vi "Shooting Managment.vi"(0 "Start Shooting Procedure":bool) -> (1 "Disable Stack Ordering":bool, 2 "Is Shooting?":bool)   [LabVIEW 2012]
uses:
  BotStatus.vi
panel:
  # "ADD Override!!!!!!!!!!!!!!!!!!!!!!!!"
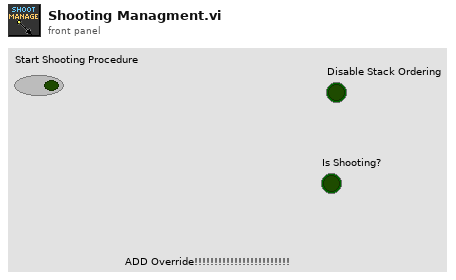
[diagram p1: front panel]
types:
  T1 = cluster{"Middle":bool, "Cannon":bool, "InFlipper":bool, "FlipperAtPlace":bool, "Bottom":bool, "FrisbeeDirection":bool}
  T2 = typedef "WPI_MotorControlDeviceRef.ctl" = cluster{"DeviceStatus":errorcluster, "Type":enum16{"PWM", "CAN"}, "PWM":cluster{"Digital Module":T3, "PWM Channel":T4, "DeadBand":T5}, "CAN":cluster{"Device Number":u8, "Control Mode":T6, "Semaphore":T7, "Max Vout":dbl}, "Invert":bool, "TransformRef":T8, "InvTransformRef":T8}
  T3 = typedef "FPGA_TypedefDigitalModule.ctl" = enum16{"Digital Module 1", "Digital Module 2"}
  T4 = typedef "FPGA_DIOPWMChannel.ctl" = enum8{"PWM 1", "PWM 2", "PWM 3", "PWM 4", "PWM 5", "PWM 6", "PWM 7", "PWM 8", "PWM 9", "PWM 10", "Invalid"}
  T5 = typedef "WPI_PWMDeadband.ctl" = cluster{"Name":string, "maxPositivePwm":i32, "minPositivePwm":i32, "centerPwm":i32, "maxNegativePwm":i32, "minNegativePwm":i32, "angularRange":u16}
  T6 = typedef "WPI_CANJaguar_ControlMode.ctl" = enum8{"Percent VBus", "Current", "Speed", "Position", "Voltage"}
  T7 = typedef "Semaphore RefNum" = refnum<k1>
  T8 = typedef "WPI_PWMTransform_ConPane.ctl" = refnum<vi>
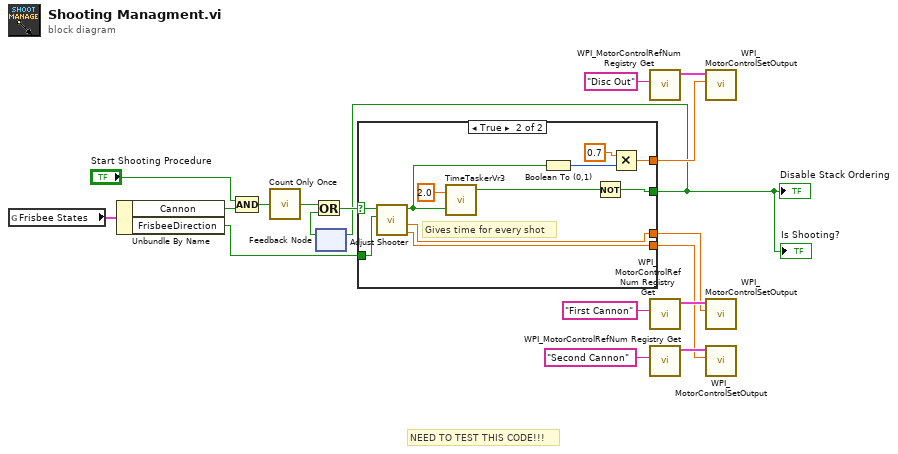
[diagram p0: block diagram]
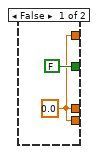
[diagram p2: hidden frame]
diagram:
  # "NEED TO TEST THIS CODE!!!"
  n1 = global read "BotStatus.vi" "Frisbee States"() -> (w5:T1)
  n2 = Unbundle By Name(w5) -> ("Cannon"=w3:bool, "FrisbeeDirection"=w4:bool)
  n3 = Compound Arithmetic op=AND("Start Shooting Procedure", w3) -> (w2:bool)
  n4 = call "Count Only Once.vi"("InValue"=w2) -> ("Result"=w17:bool)
  n5 = feedback #1() -> (w16:bool)  [unwired: 1 in]
  n6 = Or(x=w17, y=w16) -> (x .or. y?=w18:bool)
  n7 = case shown="True" w18 {
    selector: w18 -> [_ w24]
    tunnel: [FALSE ("READY!") w25] -> w1
    tunnel: [w19 w29] -> w13
    tunnel: [w19 w23] -> w8
    tunnel: [w19 w22] -> w7
    tunnel: w4 -> [_ w21]
    frame False {
      w19 = 0.0
    }
    frame True {
      # "Gives time for every shot"
      n8 = call "Adjust Shooter.vi"("Upside Down?"=w21, "Start to Adjust"=w24) -> ("Second Cannon"=w22:dbl, "First Cannon"=w23:dbl, "READY!"=w27:bool)  [unwired: 2 in, 1 out]
      n9 = call "TimeTaskerVr3.vi"("Delay(sec)"=2.0, "Start Counting?"=w27) -> ("TimePast?"=w26:bool)  [unwired: 2 out]
      n10 = Boolean To (0,1)(Boolean=w27) -> (0, 1=w31:i16)
      n11 = Not(x=w26) -> (.not. x?=w25:bool)
      n12 = Multiply(x=0.7, y=w31) -> (x*y=w29:dbl)
    }
  }
  "Disable Stack Ordering" <- w1
  "Is Shooting?" <- w1
  n13 = feedback-in #1(w1) -> ()
  n14 = call <vilib>:"WPI_MotorControlRefNum Registry Get.vi"("refnum name"="Disc Out") -> ("MotorControlDevRef"=w15:T2)  [unwired: 9 in, 1 out]
  n15 = call <vilib>:"WPI_MotorControlRefNum Registry Get.vi"("refnum name"="First Cannon") -> ("MotorControlDevRef"=w12:T2)  [unwired: 9 in, 1 out]
  n16 = call <vilib>:"WPI_MotorControlRefNum Registry Get.vi"("refnum name"="Second Cannon") -> ("MotorControlDevRef"=w11:T2)  [unwired: 9 in, 1 out]
  n17 = call <vilib>:"WPI_MotorControlSetOutput.vi"("Output"=w13, "MotorControlDevRef"=w15) -> ()  [unwired: 7 in, 3 out]
  n18 = call <vilib>:"WPI_MotorControlSetOutput.vi"("Output"=w8, "MotorControlDevRef"=w12) -> ()  [unwired: 7 in, 3 out]
  n19 = call <vilib>:"WPI_MotorControlSetOutput.vi"("Output"=w7, "MotorControlDevRef"=w11) -> ()  [unwired: 7 in, 3 out]
